vi "Python_Interface.vi"() -> ()   [LabVIEW 2022 SP3]
panel:
  in  "Python path":path
  out "String 2":string
  in  "String":string
  in  "Python version":string
  in  "function name":string
  in  "module path":path
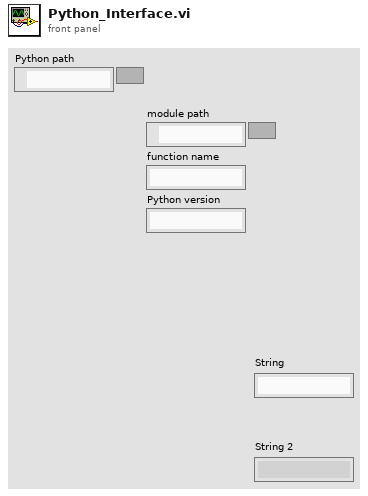
[diagram p1: front panel]
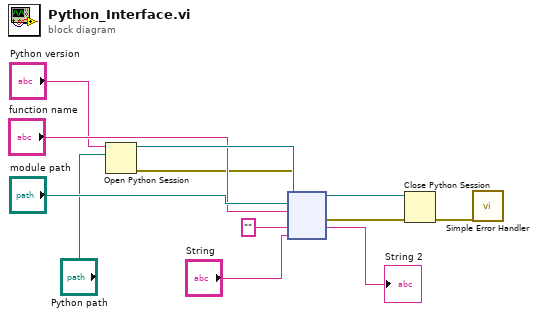
[diagram p0: block diagram]
diagram:
  n1 = Open Python Session(python version="Python version", python path="Python path") -> (session out=w12:refnum<k35>, error out=w5:errorcluster)  [unwired: 1 in]
  n2 = node(w12, "module path", "function name", w5, "", "String") -> (w11:refnum<k35>, w10:errorcluster, →"String 2":string)  [unwired: 1 in, 2 out]
  n3 = Close Python Session(session in=w11, error in=w10) -> (11:w6:errorcluster)
  n4 = call <vilib>:"Simple Error Handler.vi"("error in (no error)"=w6) -> ()  [unwired: 4 in, 5 out]
